vi "get_numeric_type_info.vi"(8 "error in (no error)":errorcluster, 10 "Refnum":refnum<vi>) -> (0 "error out":errorcluster, 1 "Precision":string, 2 "max":string, 3 "Min":string)   [LabVIEW 2020]
panel:
  in  "DummyNumeric 2":refnum<vi>
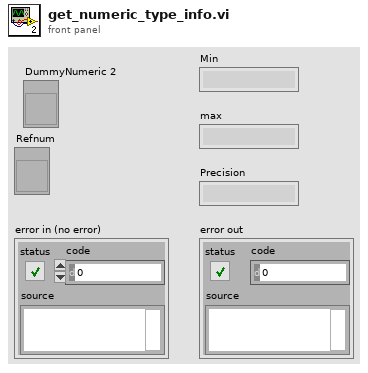
[diagram p1: front panel]
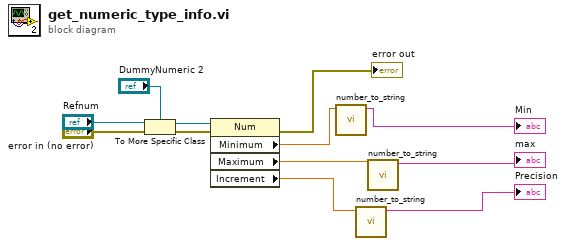
[diagram p0: block diagram]
diagram:
  n1 = To More Specific Class(target class="DummyNumeric 2", reference="Refnum", error in="error in (no error)") -> (specific class reference=w12:refnum<vi>, error out=w9:errorcluster)
  n2 = property class="Num"(reference=w12, error in=w9) -> (error out=→"error out":errorcluster, "Minimum"=w5:dbl, "Maximum"=w2:dbl, "Increment"=w4:dbl)  [unwired: 1 out]
  n3 = call "number_to_string.vi"("input 1"=w5) -> ("String"=→"Min":string)  [unwired: 10 in]
  n4 = call "number_to_string.vi"("input 1"=w4) -> ("String"=→"Precision":string)  [unwired: 10 in]
  n5 = call "number_to_string.vi"("input 1"=w2) -> ("String"=→"max":string)  [unwired: 10 in]
